vi "NI9205_SUB-VI_INIT.vi"(7 "SampleRate":dbl, 8 "error in (no error)":errorcluster, 9 "MaximumSampleRate?":bool, 10 "Channels NI9205":tag, 11 "Number of Samples":i32) -> (0 "error out":errorcluster, 1 "SampQuant.SampPerChan":dbl, 2 "SampClk.MaxRate":dbl, 3 "Refnum out":refnum<k21>)   [LabVIEW 2020]
uses:
  <vilib>/DAQmx/create/channels.llb/DAQmx Create Channel (AI-Voltage-Basic).vi
  <vilib>/DAQmx/configure/timing.llb/DAQmx Timing (Sample Clock).vi
  <resource>/objmgr/daqmx.rc
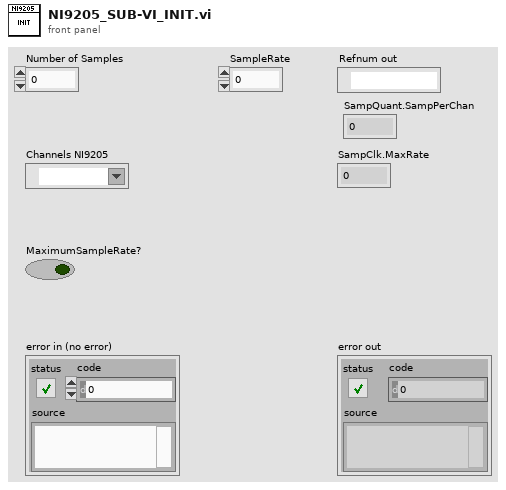
[diagram p1: front panel]
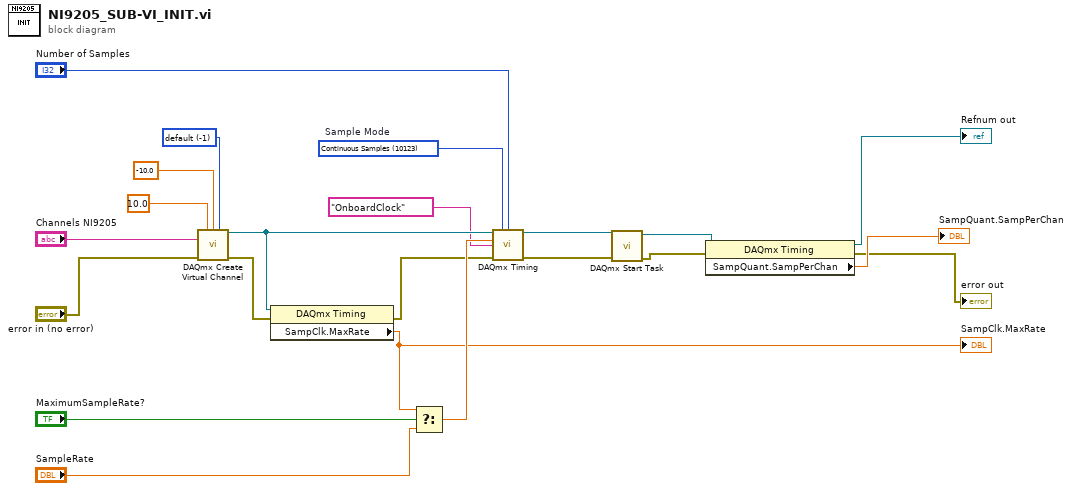
[diagram p0: block diagram]
diagram:
  w9 = -1 items=["default"=-1, "RSE"=10083, "NRSE"=10078, "Differential"=10106, "Pseudodifferential"=12529] ("Terminal Configuration")
  w8 = 10123 items=["Finite Samples"=10178, "Continuous Samples"=10123, "Hardware Timed Single Point"=12522]  # Sample Mode
  n1 = call-poly <vilib>:"DAQmx Create Virtual Channel.vi"("maximum value"=10.0 ("Max Voltage"), "minimum value"=-10.0 ("Min Voltage"), "input terminal configuration"=w9, "physical channels"="Channels NI9205", "error in"="error in (no error)") -> ("task out"=w17:refnum<k21>, "error out"=w2:errorcluster)  [unwired: 9 in]
  n2 = property class="DAQmx Timing"(reference=w17, error in=w2) -> (error out=w1:errorcluster, "SampClk.MaxRate"=w20:dbl)  [unwired: 1 out]
  "SampClk.MaxRate" <- w20
  n3 = Select(t=w20, s="MaximumSampleRate?", f="SampleRate") -> (s? t:f=w22:dbl)
  n4 = call-poly <vilib>:"DAQmx Timing.vi"("task/channels in"=w17, "sample mode"=w8, "samples per channel"="Number of Samples", "rate"=w22, "source"=tag "OnboardClock" ("Sample Clock Source"), "error in"=w1) -> ("task out"=w16:refnum<k21>, "error out"=w13:errorcluster)  [unwired: 8 in]
  n5 = call <vilib>:"DAQmx Start Task.vi"("task/channels in"=w16, "error in"=w13) -> ("task out"=w7:refnum<k21>, "error out"=w5:errorcluster)  [unwired: 12 in]
  n6 = property class="DAQmx Timing"(reference=w7, error in=w5) -> (reference out=→"Refnum out":refnum<k21>, error out=→"error out":errorcluster, "SampQuant.SampPerChan"=→"SampQuant.SampPerChan":dbl)
